vi "test-SwerveDrvPoseEst2-Test1.vi"(8 "error in (no error)":errorcluster) -> (0 "error out":errorcluster, 3 "Test Passed":bool)   [LabVIEW 2019]
uses:
  <vilib>/Rock Robotics/WPI/ThirdParty/JAS_Junk/TrajLib/Trajectory_Library.lvlib
panel:
  out "Sub error":bool
  out "End Y pos passed":bool
  out "End X pos passed":bool
  out "AddVisionCount":i32
  out "TotalTImeSecs 2":dbl
  out "BenchProcessing \nTimer Per Pass":dbl
  out "BenchTotalTime":dbl
  out "BenchTotalPasses":dbl
  out "MaxErrPassed":bool
  out "MeanPassed":bool
  out "ErrorSumNormalized":dbl
  out "Error Sum":dbl
  out "Max Error":dbl
  out "VIsionMeasCount":i32
  out "TotalTImeSecs":dbl
  out "Position Graph":cluster{dbl[], dbl[]}[](graph)
  out "PoseEst2NewErr":errorcluster
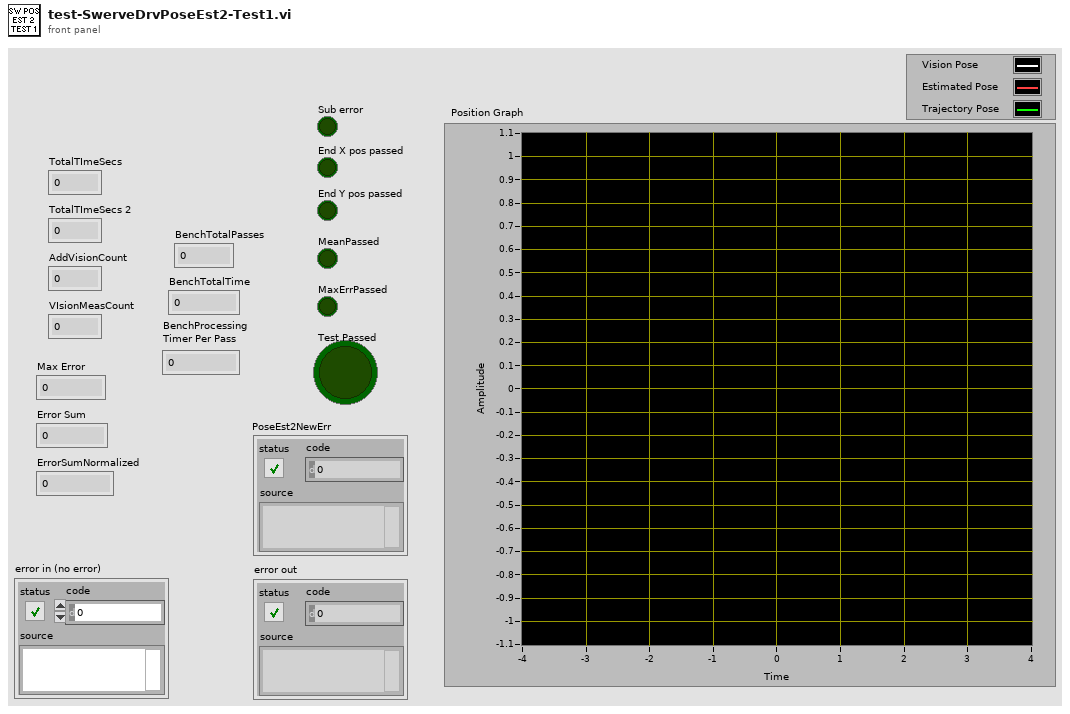
[diagram p1: front panel]
types:
  T1 = typedef "Trajectory_Library.lvlib/TRANSLATION2D.ctl" = cluster{"X":dbl, "Y":dbl}
  T2 = typedef "Trajectory_Library.lvlib/ROTATION2D.ctl" = cluster{"VALUE":dbl, "COS":dbl, "SIN":dbl}
  T3 = typedef "Trajectory_Library.lvlib/SWERVE_DRIVE_MODULE_POSITION.ctl" = cluster{"Distance":dbl, "Angle":T2, "P":bool}
  T4 = typedef "Trajectory_Library.lvlib/SWERVE_DRIVE_KINEMATICS.ctl" = cluster{"NumModules":i32, "InverseKinematics":T5, "ForwardKinematics":T5, "Modules":T1[], "PrevCoR":T1, "SavedModuleStates":T6[]}
  T5 = typedef "NI_Matrix.lvlib/RealMatrix.ctl" = dbl[][]
  T6 = typedef "Trajectory_Library.lvlib/SWERVE_DRIVE_MODULE_STATE.ctl" = cluster{"Speed":dbl, "Angle":T2}
  T7 = typedef "Trajectory_Library.lvlib/POSE2D.ctl" = cluster{"TRANSLATION":T1, "ROTATION":T2}
  T8 = typedef "Trajectory_Library.lvlib/TRAJ_CONFIG.ctl" = cluster{"MaxVelocity":dbl, "Max Acceleration":dbl, "StartVelocity":dbl, "End Velocity":dbl, "Reversed":bool, "Constraints":variant[]}
  T9 = typedef "Trajectory_Library.lvlib/SWERVE_DRIVE_POSE_EST2.ctl" = cluster{"M_Vision_K":T5, "m_nominal_dT":dbl, "m_PrevTime_Sec":dbl, "Pose_Buffer":T10, "Swerve_Drive_Kinematics":T4, "Swerve_Drive_Odom":T11, "M_Q":T5, "NumModules":i32}
  T10 = typedef "Trajectory_Library.lvlib/TIME_INTERPOLATABLE_VARIANT.ctl" = cluster{"TimeStamps":dbl[], "DataArray":variant[], "Min_TimeStamp":dbl, "Max_TimeStamp":dbl, "ItemCount":i32, "MaxBufferTime":dbl}
  T11 = typedef "Trajectory_Library.lvlib/SWERVE_DRIVE_ODOMETRY.ctl" = cluster{"POSE":T7, "GyroOffset":T2, "PreviousAngle":T2, "PrevModulePositions":T3[], "NumModules":i32}
  T12 = typedef "Trajectory_Library.lvlib/TRAJECTORY.ctl" = cluster{"TotalTImeSecs":dbl, "States":T13[]}
  T13 = typedef "Trajectory_Library.lvlib/TRAJ_STATE.ctl" = cluster{"TimeSeconds":dbl, "Velocity":dbl, "Acceleration":dbl, "POSE":T7, "Curvature":dbl}
  T14 = cluster{"MaxErrPassed":bool, "MeanPassed":bool, "Error Sum":dbl, "ErrorSumNormalized":dbl, "Max Error":dbl, "AddVisionCount":i32, "VIsionApplyCount":i32, "BenchTotalPasses":dbl, "BenchTotalTime":dbl, "BenchProcessing \nTimer Per Pass":dbl, "TotalTImeSecs":dbl, "End X pos passed":bool, "End Y pos passed":bool, "Sub error":bool, "End X Dev":dbl, "End Y Dev":dbl}
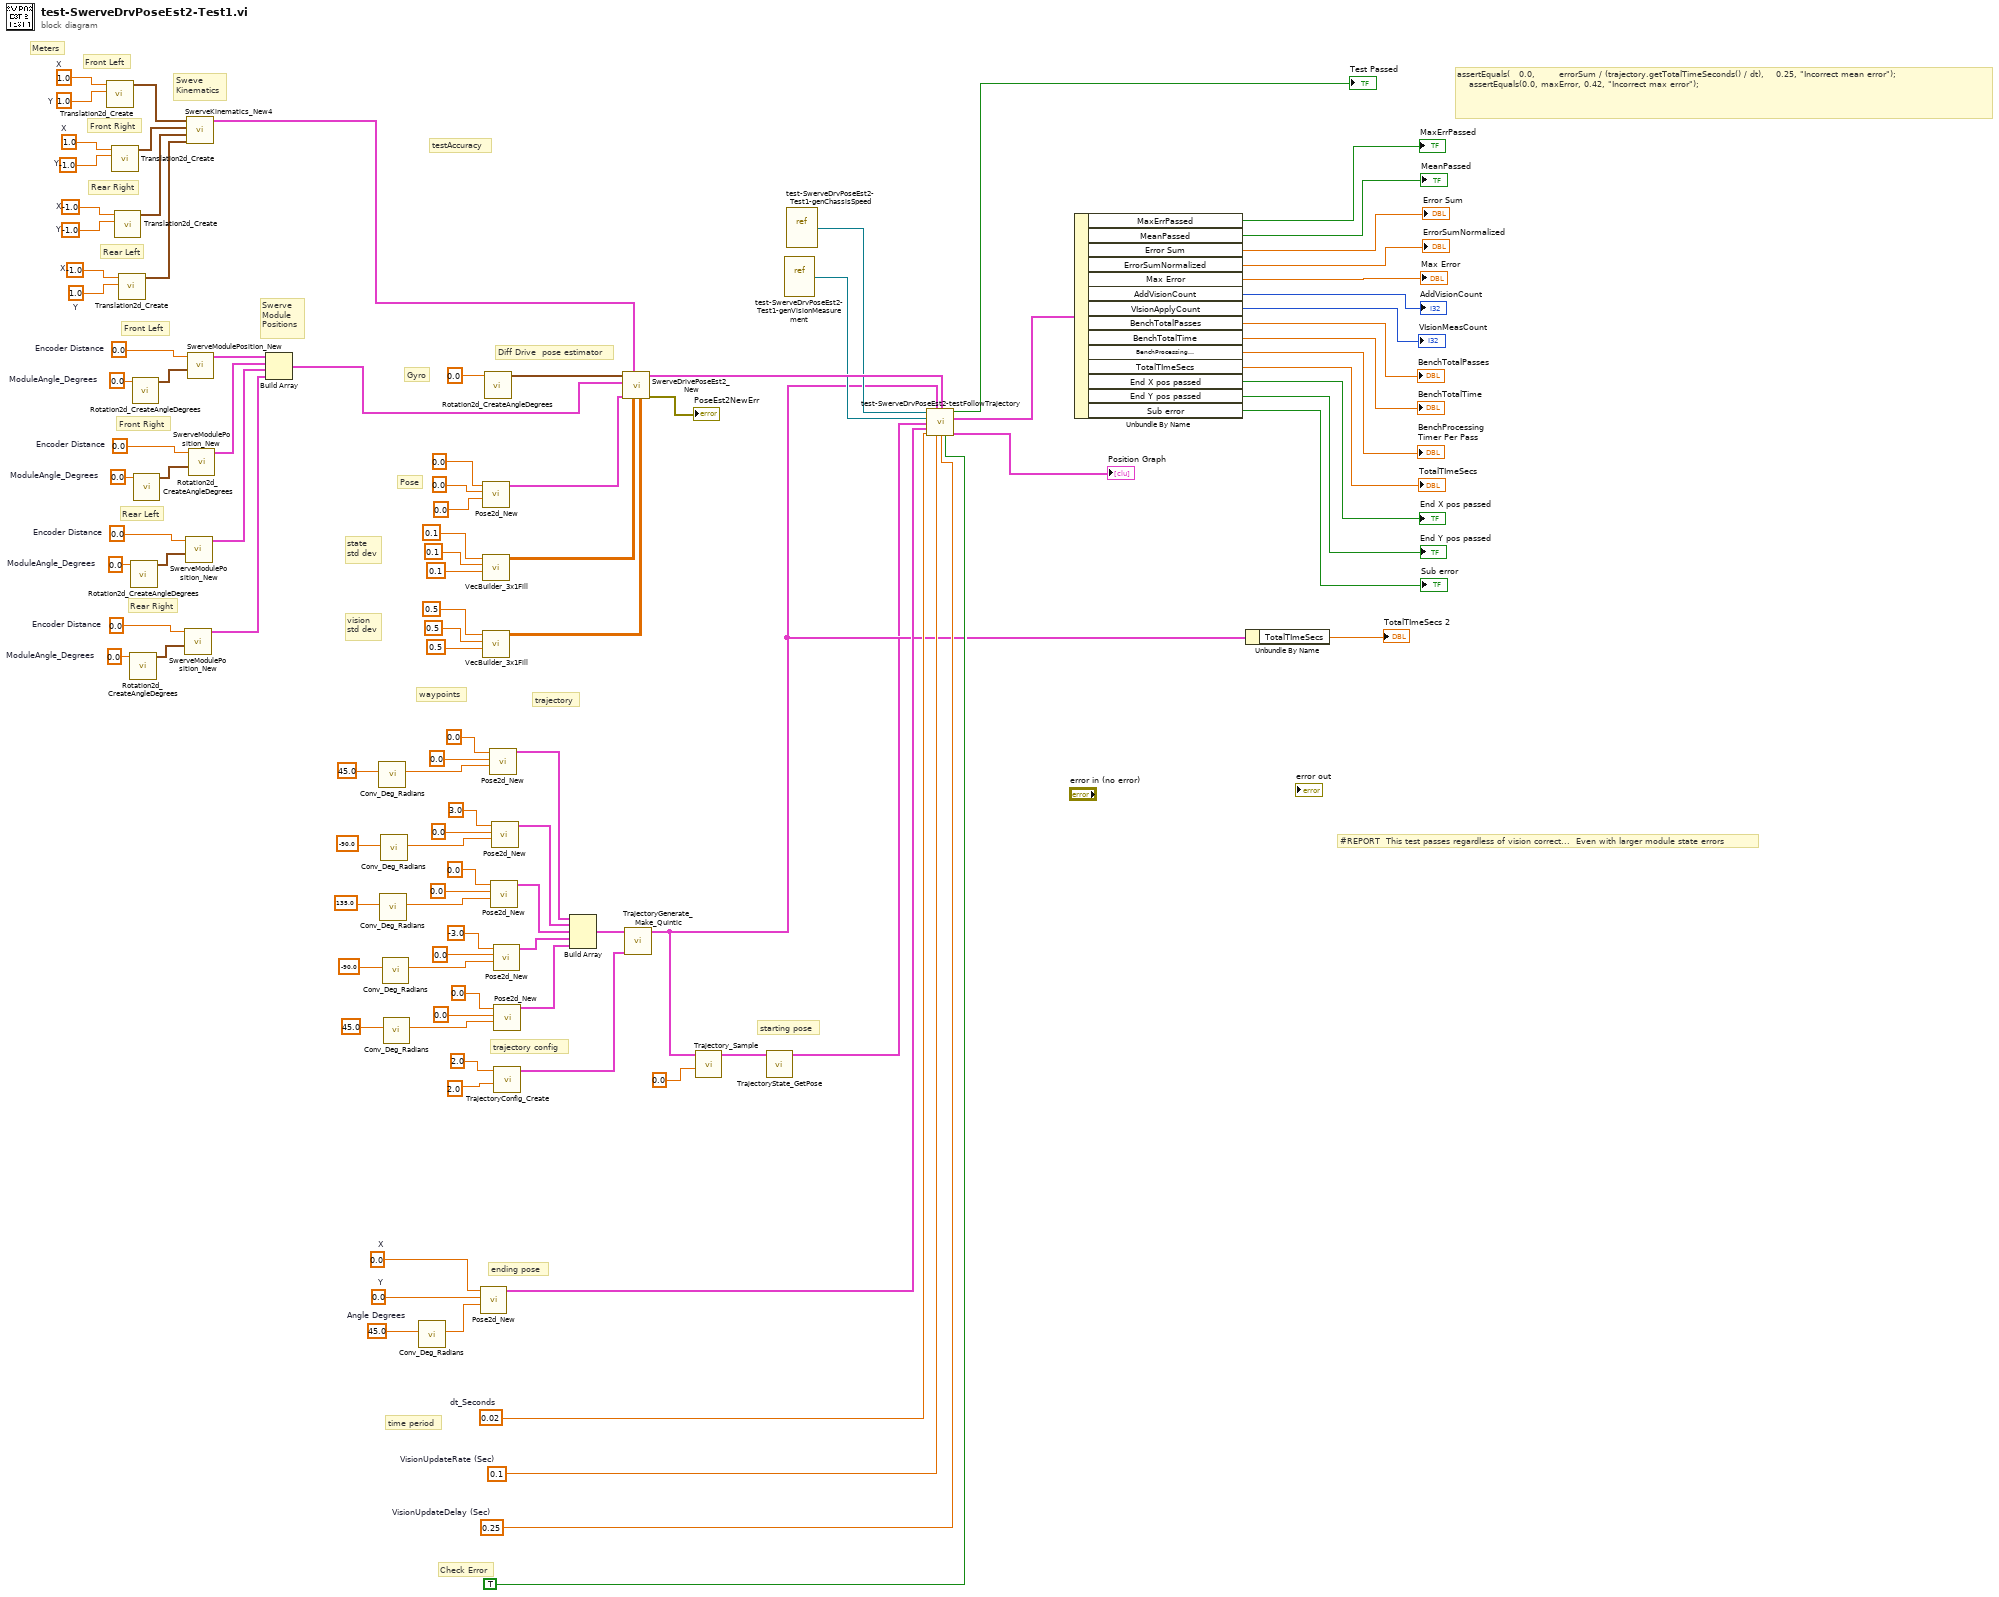
[diagram p0: block diagram]
diagram:
  w9 = -1.0  # X
  w8 = 1.0  # Y
  w7 = -1.0  # X
  w6 = -1.0  # Y
  w5 = 1.0  # X
  w4 = -1.0  # Y
  w3 = 1.0  # X
  w2 = 1.0  # Y
  w27 = 0.0  # ModuleAngle_Degrees
  w25 = 0.0  # Encoder Distance
  w24 = 0.0  # ModuleAngle_Degrees
  w22 = 0.0  # Encoder Distance
  w21 = 0.0  # ModuleAngle_Degrees
  w19 = 0.0  # Encoder Distance
  w17 = 0.0  # ModuleAngle_Degrees
  w15 = 0.0  # Encoder Distance
  w56 = 0.25  # VisionUpdateDelay (Sec)
  w57 = 0.1  # VisionUpdateRate (Sec)
  w62 = 0.0  # X
  w61 = 0.0  # Y
  w59 = 45.0  # Angle Degrees
  w63 = 0.02  # dt_Seconds
  # "Meters"
  # "Sweve\nKinematics"
  # "Rear Right"
  # "Rear Left"
  # "Front Right"
  # "Front Left"
  # "Front Left"
  # "Swerve\nModule\nPositions"
  # "Rear Right"
  # "Rear Left"
  # "Front Right"
  # "testAccuracy"
  # "starting pose"
  # "Check Error"
  # "ending pose"
  # "state \nstd dev"
  # "#REPORT  This test passes regardless of vision correct...  Even with larger module state errors"
  # "assertEquals(   0.0,        errorSum / (trajectory.getTotalTimeSeconds() / dt),    0.25, \"Incorrect mean error\");\n    assertEquals(0.0, maxError, 0.42, \"Incorrect max error\");"
  # "time period"
  # "vision \nstd dev"
  # "Pose"
  # "Gyro"
  # "Diff Drive  pose estimator"
  # "trajectory config"
  # "trajectory"
  # "waypoints"
  n1 = call <vilib>:"Translation2d_Create.vi"("Y"=w2, "X"=w3) -> ("TRANSLATION"=w10:T1)  [unwired: 9 in]
  n2 = call <vilib>:"Translation2d_Create.vi"("Y"=w4, "X"=w5) -> ("TRANSLATION"=w11:T1)  [unwired: 9 in]
  n3 = call <vilib>:"Translation2d_Create.vi"("Y"=w6, "X"=w7) -> ("TRANSLATION"=w12:T1)  [unwired: 9 in]
  n4 = call <vilib>:"Translation2d_Create.vi"("Y"=w8, "X"=w9) -> ("TRANSLATION"=w13:T1)  [unwired: 9 in]
  n5 = call <vilib>:"Rotation2d_CreateAngleDegrees.vi"("Angle_Degrees"=w27) -> ("ROTATION"=w26:T2)  [unwired: 10 in]
  n6 = call <vilib>:"Rotation2d_CreateAngleDegrees.vi"("Angle_Degrees"=w24) -> ("ROTATION"=w23:T2)  [unwired: 10 in]
  n7 = call <vilib>:"Rotation2d_CreateAngleDegrees.vi"("Angle_Degrees"=w17) -> ("ROTATION"=w16:T2)  [unwired: 10 in]
  n8 = call <vilib>:"Rotation2d_CreateAngleDegrees.vi"("Angle_Degrees"=w21) -> ("ROTATION"=w20:T2)  [unwired: 10 in]
  n9 = call <vilib>:"SwerveModulePosition_New.vi"("ROTATION"=w26, "Distance"=w25) -> ("SWERVE_DRIVE_MODULE_POSITION"=w30:T3)  [unwired: 9 in]
  n10 = call <vilib>:"SwerveModulePosition_New.vi"("ROTATION"=w23, "Distance"=w22) -> ("SWERVE_DRIVE_MODULE_POSITION"=w29:T3)  [unwired: 9 in]
  n11 = call <vilib>:"SwerveKinematics_New4.vi"("wheel 3"=w13, "wheel 2"=w12, "wheel 1"=w11, "wheel 0"=w10) -> ("SWERVE_DRIVE_KINEMATICS"=w1:T4)  [unwired: 7 in]
  n12 = call <vilib>:"SwerveModulePosition_New.vi"("ROTATION"=w16, "Distance"=w15) -> ("SWERVE_DRIVE_MODULE_POSITION"=w18:T3)  [unwired: 9 in]
  n13 = call <vilib>:"SwerveModulePosition_New.vi"("ROTATION"=w20, "Distance"=w19) -> ("SWERVE_DRIVE_MODULE_POSITION"=w28:T3)  [unwired: 9 in]
  n14 = Build Array(w18, w28, w29, w30) -> (w14:T3[])
  n15 = call <vilib>:"Conv_Deg_Radians.vi"("Degress"=45.0 ("Heading")) -> ("Radians"=w85:dbl)  [unwired: 10 in]
  n16 = call <vilib>:"Conv_Deg_Radians.vi"("Degress"=135.0 ("Heading")) -> ("Radians"=w93:dbl)  [unwired: 10 in]
  n17 = call <vilib>:"Conv_Deg_Radians.vi"("Degress"=-90.0 ("Heading")) -> ("Radians"=w89:dbl)  [unwired: 10 in]
  n18 = call <vilib>:"Conv_Deg_Radians.vi"("Degress"=-90.0 ("Heading")) -> ("Radians"=w97:dbl)  [unwired: 10 in]
  n19 = call <vilib>:"Conv_Deg_Radians.vi"("Degress"=45.0 ("Heading")) -> ("Radians"=w101:dbl)  [unwired: 10 in]
  n20 = call <vilib>:"Conv_Deg_Radians.vi"("Degress"=w59) -> ("Radians"=w60:dbl)  [unwired: 10 in]
  n21 = call <vilib>:"Pose2d_New.vi"("Heading"=w60, "Y"=w61, "X"=w62) -> ("out POSe"=w58:T7)  [unwired: 8 in]
  n22 = call <vilib>:"Pose2d_New.vi"("Heading"=0.0, "Y"=0.0, "X"=0.0) -> ("out POSe"=w71:T7)  [unwired: 8 in]
  n23 = call <vilib>:"VecBuilder_3x1Fill.vi"("R2"=0.1 ("element"), "R1"=0.1 ("element"), "R0"=0.1 ("element")) -> ("output matrix"=w66:T5)  [unwired: 8 in]
  n24 = call <vilib>:"VecBuilder_3x1Fill.vi"("R2"=0.5 ("element"), "R1"=0.5 ("element"), "R0"=0.5 ("element")) -> ("output matrix"=w65:T5)  [unwired: 8 in]
  n25 = call <vilib>:"Rotation2d_CreateAngleDegrees.vi"("Angle_Degrees"=0.0) -> ("ROTATION"=w70:T2)  [unwired: 10 in]
  n26 = call <vilib>:"Pose2d_New.vi"("Heading"=w85, "Y"=0.0, "X"=0.0) -> ("out POSe"=w84:T7)  [unwired: 8 in]
  n27 = call <vilib>:"Pose2d_New.vi"("Heading"=w93, "Y"=0.0, "X"=0.0) -> ("out POSe"=w81:T7)  [unwired: 8 in]
  n28 = call <vilib>:"Pose2d_New.vi"("Heading"=w89, "Y"=0.0, "X"=3.0) -> ("out POSe"=w82:T7)  [unwired: 8 in]
  n29 = call <vilib>:"Pose2d_New.vi"("Heading"=w97, "Y"=0.0, "X"=-3.0) -> ("out POSe"=w80:T7)  [unwired: 8 in]
  n30 = call <vilib>:"Pose2d_New.vi"("Heading"=w101, "Y"=0.0, "X"=0.0) -> ("out POSe"=w106:T7)  [unwired: 8 in]
  n31 = call <vilib>:"TrajectoryConfig_Create.vi"("MaxAcceleration"=2.0, "MaxVelocity"=2.0) -> ("TRAJECTORY_CONFIG"=w103:T8)  [unwired: 9 in]
  n32 = Build Array(w84, w82, w81, w80, w106) -> (w104:T7[])
  n33 = call <vilib>:"SwerveDrivePoseEst2_New.vi"("VisionMeasurementStdDevs"=w65, "StateStdDevs"=w66, "SWERVE_DRIVE_KINEMATICS"=w1, "InitialPose"=w71, "Module Positions"=w14, "gyroAngle"=w70) -> ("Error"=→"PoseEst2NewErr":errorcluster, "SwerveDrivePoseEstimate"=w64:T9)  [unwired: 4 in]
  n34 = call <vilib>:"TrajectoryGenerate_Make_Quintic.vi"("traj_config"=w103, "waypointPOSE"=w104) -> ("TRAJECTORY"=w35:T12)  [unwired: 8 in, 1 out]
  n35 = call <vilib>:"Trajectory_Sample.vi"("Time"=0.0, "InputTRAJECTORY"=w35) -> ("OutputTRAJ_STATE"=w33:T13)  [unwired: 9 in]
  n36 = call <vilib>:"TrajectoryState_GetPose.vi"("TRAJ_STATE"=w33) -> ("TrajStatePose"=w32:T7)  [unwired: 10 in]
  n37 = vi-ref "test-SwerveDrvPoseEst2-Test1-genVisionMeasurement.vi"() -> (w52:refnum<vi>)
  n38 = vi-ref "test-SwerveDrvPoseEst2-Test1-genChassisSpeed.vi"() -> (w53:refnum<vi>)
  n39 = call "test-SwerveDrvPoseEst2-testFollowTrajectory.vi"("chassisSpeedsGenerator"=w53, "TRAJECTORY"=w35, "SwerveDrivePoseEstimate2"=w64, "genVisionMeasurement"=w52, "StartingPose"=w32, "EndingPose"=w58, "dt_Seconds"=w63, "VisionUpdateRate"=w57, "VisionUpdateDelay"=w56, "CheckError"=TRUE) -> ("Test Passed"=→"Test Passed":bool, "Output Data"=w49:T14, "DataForGraph"=→"Position Graph":cluster{dbl[], dbl[]}[])  [unwired: 3 in]
  n40 = Unbundle By Name(w49) -> ("MaxErrPassed"=→"MaxErrPassed":bool, "MeanPassed"=→"MeanPassed":bool, "Error Sum"=→"Error Sum":dbl, "ErrorSumNormalized"=→"ErrorSumNormalized":dbl, "Max Error"=→"Max Error":dbl, "AddVisionCount"=→"AddVisionCount":i32, "VIsionApplyCount"=→"VIsionMeasCount":i32, "BenchTotalPasses"=→"BenchTotalPasses":dbl, "BenchTotalTime"=→"BenchTotalTime":dbl, "BenchProcessing \nTimer Per Pass"=→"BenchProcessing \nTimer Per Pass":dbl, "TotalTImeSecs"=→"TotalTImeSecs":dbl, "End X pos passed"=→"End X pos passed":bool, "End Y pos passed"=→"End Y pos passed":bool, "Sub error"=→"Sub error":bool)
  n41 = Unbundle By Name(w35) -> ("TotalTImeSecs"=→"TotalTImeSecs 2":dbl)
